vi "Set Force Cmd Bytes.vi"(10 "ForceCmdBytes":i32, 11 "DesktopModbus in":refnum<class "DesktopModbus.lvclass">) -> (3 "DesktopModbus out":refnum<class "DesktopModbus.lvclass">)   [LabVIEW 2016]
uses:
  DesktopModbus.lvclass
  C:/CODE/ts_HPMT/Common_RT_Modbus/IModbus/IModbus.lvclass
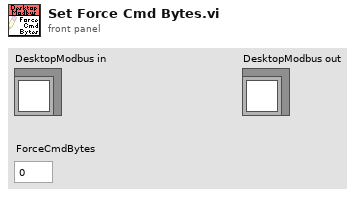
[diagram p1: front panel]
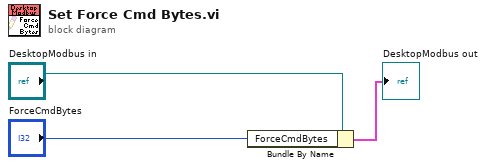
[diagram p0: block diagram]
diagram:
  n1 = Bundle By Name(cluster="DesktopModbus in", "ForceCmdBytes"="ForceCmdBytes") -> (→"DesktopModbus out":cluster{})
